vi "find_envelope.vi"(6 "lower_happen_time":dbl[](array[numeric]), 7 "lower_peak":dbl[](array[numeric]), 9 "original signal":dbl[](array[numeric]), 10 "upper_happen_time":dbl[](array[numeric]), 11 "upper_peak":dbl[](array[numeric])) -> (0 "every_mean_points":dbl[](array[numeric]), 1 "envelope_line":cluster{"xi used":dbl[], "yi":dbl[]}[](array[cluster]), 2 "lower_envelope_points":dbl[](array[numeric]), 3 "upper_envelope_points":dbl[](array[numeric]))   [LabVIEW 2018]
uses:
  <vilib>/gmath/NI_Gmath.lvlib
panel:
  out "Waveform Graph 2":dbl[](graph)
  out "Waveform Graph":dbl[](graph)
  out "upper_happen_time 2":dbl[](array[numeric])
  out "upper_peak 2":dbl[](array[numeric])
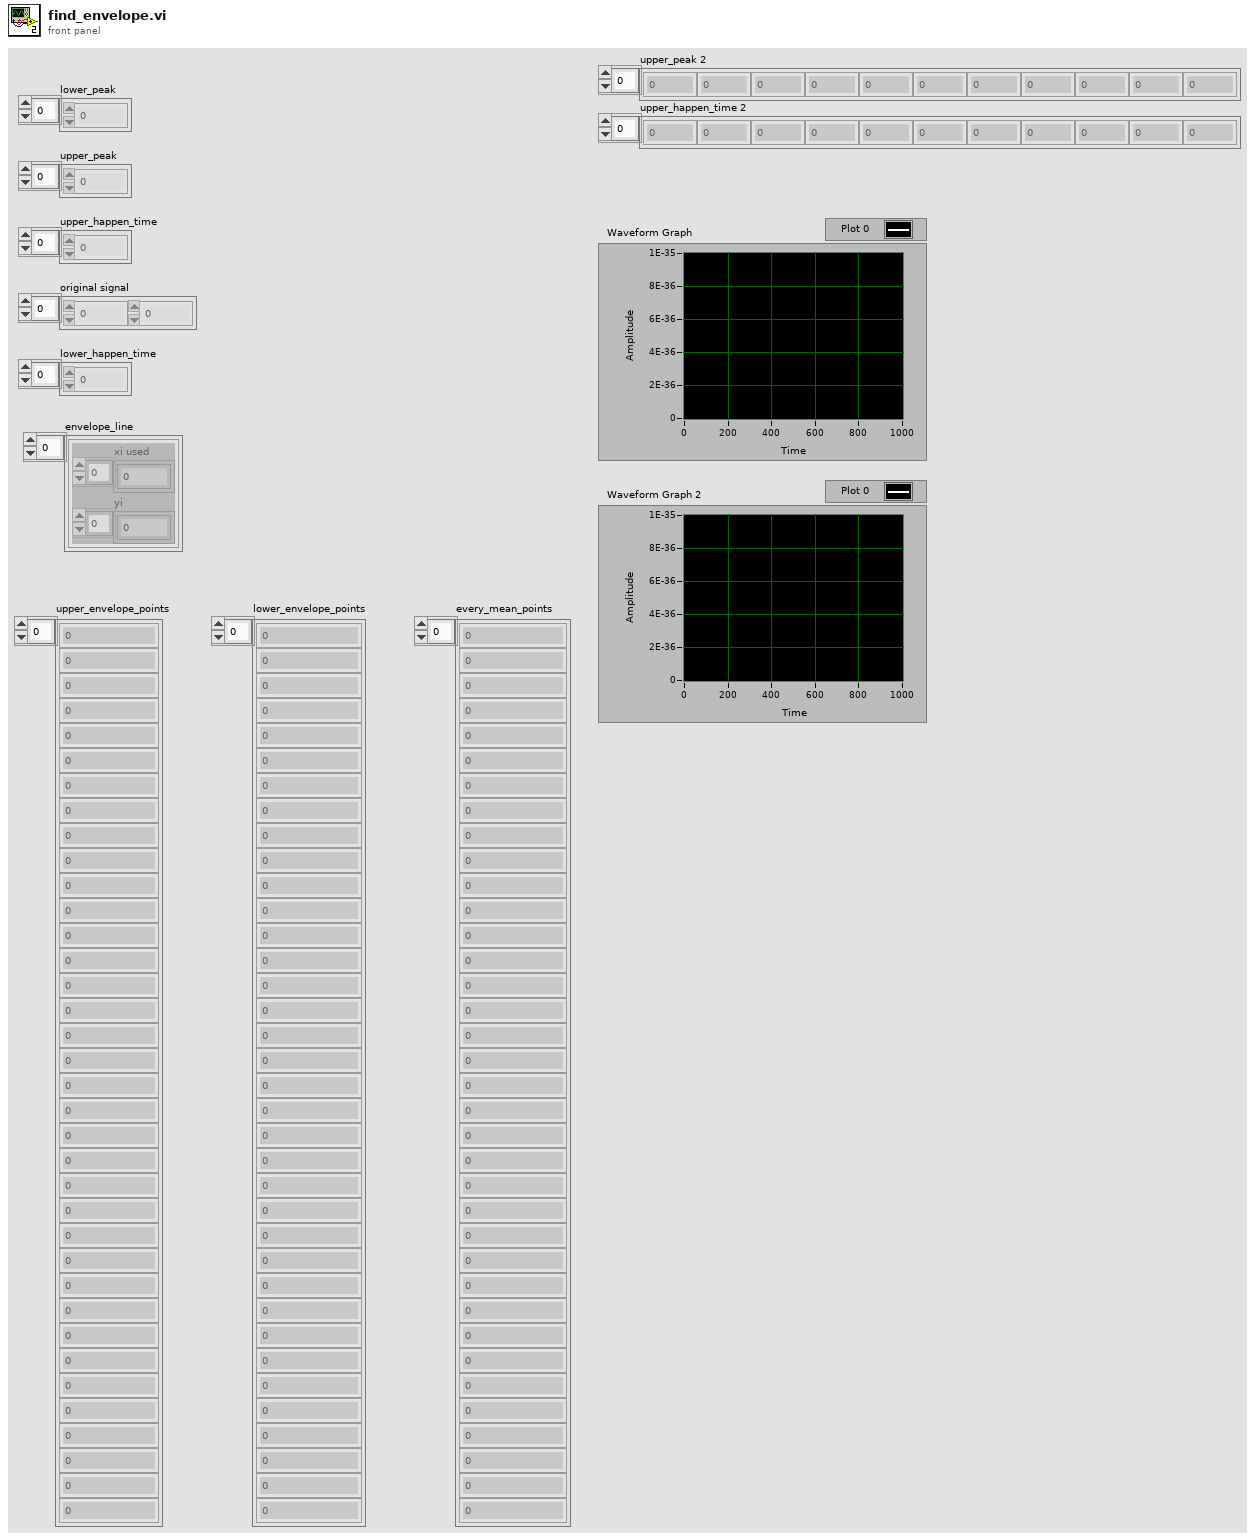
[diagram p1: front panel]
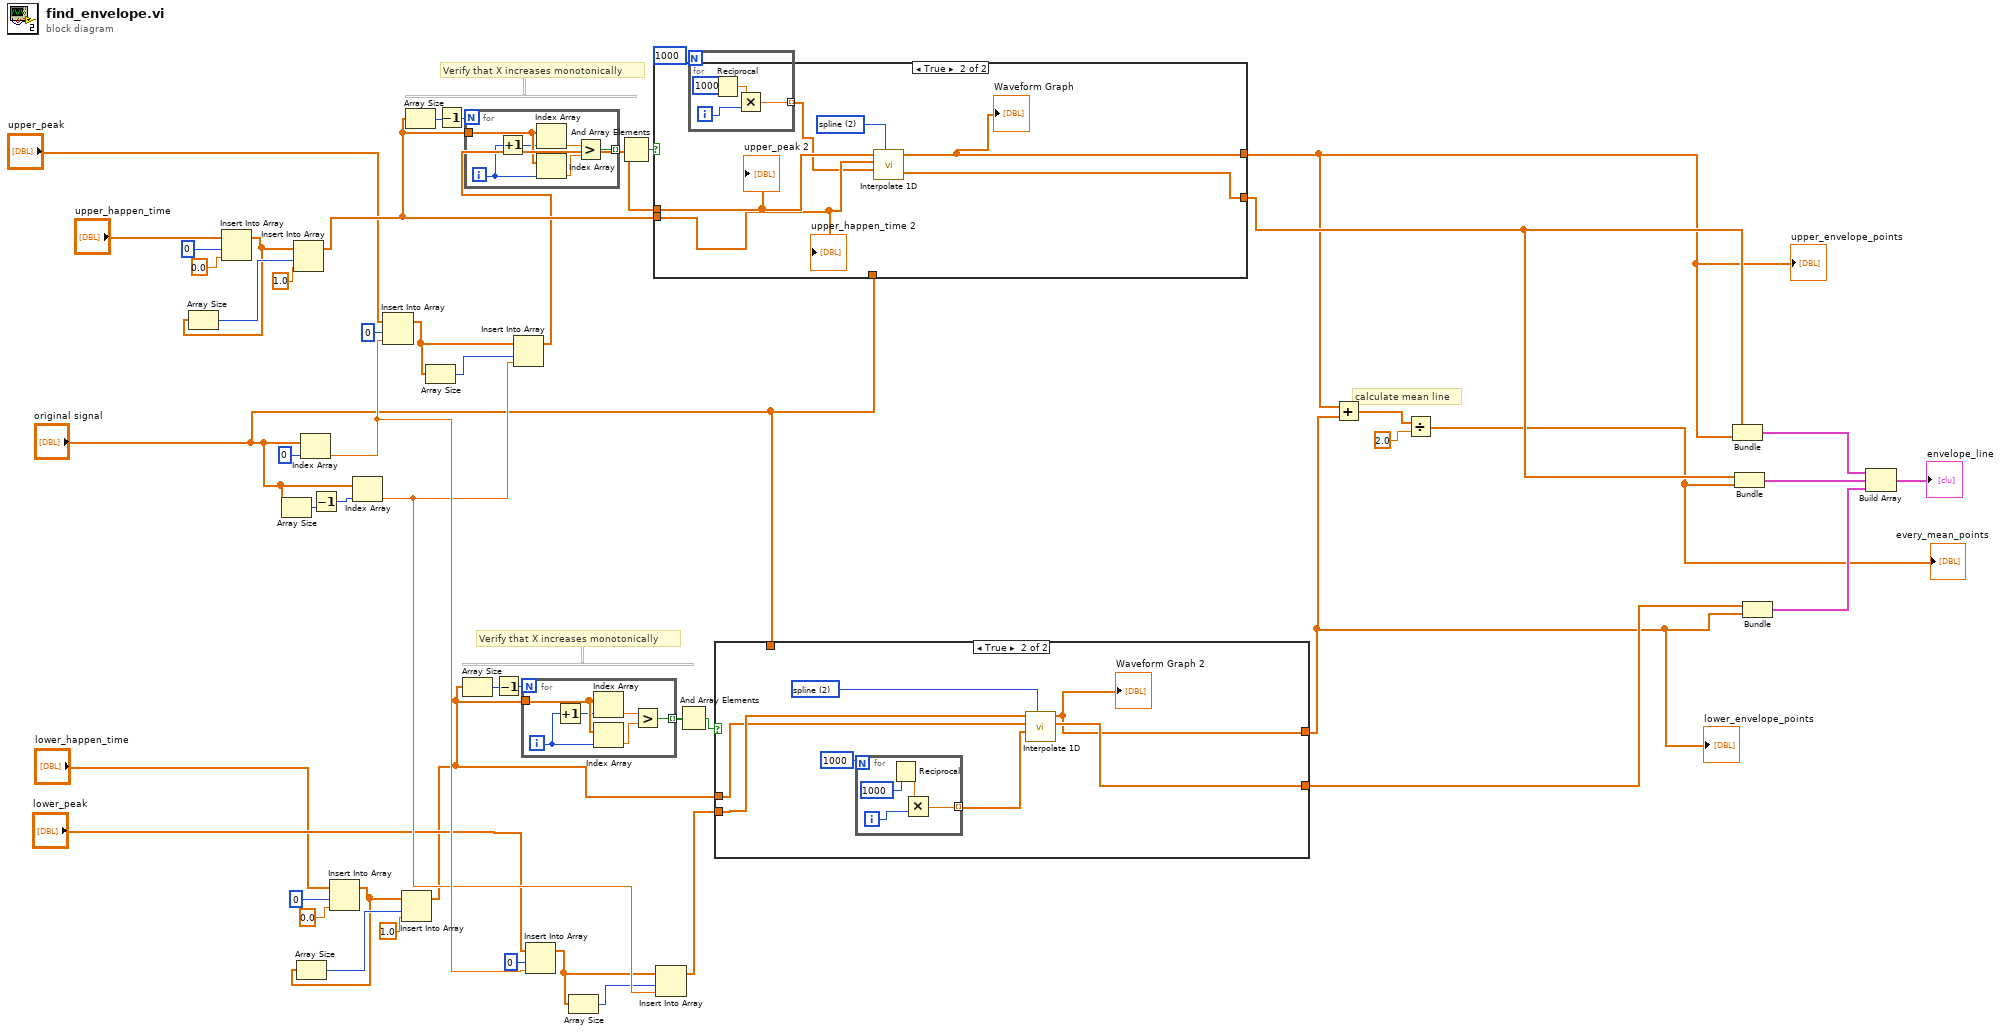
[diagram p0: block diagram]
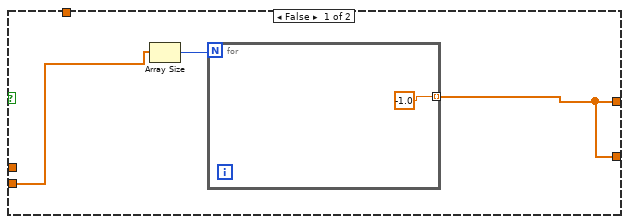
[diagram p2: hidden frame]
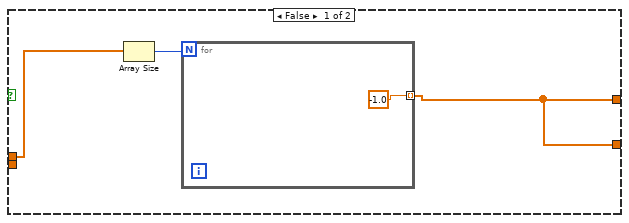
[diagram p3: hidden frame]
diagram:
  # "calculate mean line"
  # "Verify that X increases monotonically"
  # "Verify that X increases monotonically"
  n1 = Insert Into Array(array="upper_happen_time", index=0, new element=0.0 ("new element/subarray")) -> (w28:dbl[])
  n2 = Array Size(array=w28) -> (size(s)=w29:i32)
  n3 = Array Size(array="original signal") -> (size(s)=w26:i32)
  n4 = Insert Into Array(array=w28, index=w29, new element=1.0 ("new element/subarray")) -> (w34:dbl[])
  n5 = Index Array(array="original signal", index=0) -> (element=w48:dbl)
  n6 = Decrement(x=w26) -> (x-1=w25:i32)
  n7 = Insert Into Array(array="lower_happen_time", index=0, new element=0.0 ("new element/subarray")) -> (w35:dbl[])
  n8 = Array Size(array=w35) -> (size(s)=w36:i32)
  n9 = Index Array(array="original signal", index=w25) -> (element=w47:dbl)
  n10 = Insert Into Array(array="upper_peak", index=0, new element=w48) -> (w21:dbl[])
  n11 = Insert Into Array(array=w35, index=w36, new element=1.0 ("new element/subarray")) -> (w41:dbl[])
  n12 = Array Size(array=w34) -> (size(s)=w17:i32)
  n13 = Array Size(array=w21) -> (size(s)=w20:i32)
  n14 = Decrement(x=w17) -> (x-1=w16:i32)
  n15 = Array Size(array=w41) -> (size(s)=w13:i32)
  n16 = for {
    N: w16 -> [_]
    tunnel: w34 -> [w55]
    tunnel: [w50] -> w15 mode=indexing
    i -> [w53]
    n17 = Increment(x=w53) -> (x+1=w54:i32)
    n18 = Index Array(array=w55, index=w54) -> (element=w52:dbl)
    n19 = Index Array(array=w55, index=w53) -> (element=w51:dbl)
    n20 = Greater?(x=w52, y=w51) -> (0:w50:bool)
  }
  n21 = Decrement(x=w13) -> (x-1=w12:i32)
  n22 = Insert Into Array(array=w21, index=w20, new element=w47) -> (w24:dbl[])
  n23 = for {
    N: w12 -> [_]
    tunnel: w41 -> [w61]
    tunnel: [w56] -> w11 mode=indexing
    i -> [w59]
    n24 = Increment(x=w59) -> (x+1=w60:i32)
    n25 = Index Array(array=w61, index=w60) -> (element=w58:dbl)
    n26 = Index Array(array=w61, index=w59) -> (element=w57:dbl)
    n27 = Greater?(x=w58, y=w57) -> (0:w56:bool)
  }
  n28 = Insert Into Array(array="lower_peak", index=0, new element=w48) -> (w43:dbl[])
  n29 = Array Size(array=w43) -> (size(s)=w44:i32)
  n30 = And Array Elements(Boolean array=w15) -> (logical AND=w14:bool)
  n31 = case shown="True" w14 {
    tunnel: w24 -> [w63 w70]
    tunnel: w34 -> [_ w69]
    tunnel: [w62 w66] -> w6
    tunnel: [w62 w71] -> w8
    tunnel: "original signal" -> [_ _]
    frame False {
      n32 = Array Size(array=w63) -> (size(s)=w64:i32)
      n33 = for {
        N: w64 -> [_]
        tunnel: [-1.0] -> w62 mode=indexing
      }
    }
    frame True {
      w72 = 2 items=["nearest", "linear", "spline", "cubic Hermite", "Lagrange"] ("method")
      n34 = for {
        N: 1000 -> [_]
        tunnel: [w73] -> w67 mode=indexing
        i -> [w76]
        n35 = Reciprocal(x=1000) -> (1/x=w75:dbl)
        n36 = Multiply(x=w75, y=w76) -> (x*y=w73:dbl)
      }
      n37 = call <vilib>:"Interpolate 1D.vi"("method"=w72, "xi"=w67, "X"=w69, "Y"=w70) -> ("xi used"=w71:dbl[], "yi"=w66:dbl[])  [unwired: 5 in, 1 out]
      "Waveform Graph" <- w66
      "upper_peak 2" <- w70
      "upper_happen_time 2" <- w69
    }
  }
  "upper_envelope_points" <- w6
  n38 = Insert Into Array(array=w43, index=w44, new element=w47) -> (w46:dbl[])
  n39 = And Array Elements(Boolean array=w11) -> (logical AND=w10:bool)
  n40 = case shown="True" w10 {
    tunnel: w46 -> [w78 w85]
    tunnel: w41 -> [_ w83]
    tunnel: [w77 w84] -> w4
    tunnel: [w77 w86] -> w5
    tunnel: "original signal" -> [_ _]
    frame False {
      n41 = Array Size(array=w78) -> (size(s)=w79:i32)
      n42 = for {
        N: w79 -> [_]
        tunnel: [-1.0] -> w77 mode=indexing
      }
    }
    frame True {
      w87 = 2 items=["nearest", "linear", "spline", "cubic Hermite", "Lagrange"] ("method")
      n43 = for {
        N: 1000 -> [_]
        tunnel: [w88] -> w81 mode=indexing
        i -> [w91]
        n44 = Reciprocal(x=1000) -> (1/x=w90:dbl)
        n45 = Multiply(x=w90, y=w91) -> (x*y=w88:dbl)
      }
      n46 = call <vilib>:"Interpolate 1D.vi"("method"=w87, "xi"=w81, "X"=w83, "Y"=w85) -> ("xi used"=w86:dbl[], "yi"=w84:dbl[])  [unwired: 5 in, 1 out]
      "Waveform Graph 2" <- w84
    }
  }
  "lower_envelope_points" <- w4
  n47 = Add(x=w6, y=w4) -> (x+y=w2:dbl[])
  n48 = Divide(x=w2, y=2.0) -> (x/y=w1:dbl[])
  "every_mean_points" <- w1
  n49 = Bundle("xi used"=w8, "yi"=w6) -> (w19:cluster{"xi used":dbl[], "yi":dbl[]})  [unwired: 1 in]
  n50 = Bundle("xi used"=w8, w1) -> (w7:cluster{"xi used":dbl[], dbl[]})  [unwired: 1 in]
  n51 = Bundle("xi used"=w5, "yi"=w4) -> (w49:cluster{"xi used":dbl[], "yi":dbl[]})  [unwired: 1 in]
  n52 = Build Array(w19, w7, w49) -> (→"envelope_line":cluster{"xi used":dbl[], "yi":dbl[]}[])
